vi "test2.vi"() -> ()   [LabVIEW 2009]
panel:
  out "time to read":dbl
  out "error out 2":errorcluster
  out "standard error 2":string
  out "standard output 2":string
  in  "command line 2":string
  out "time to create":dbl
  out "error out":errorcluster
  out "standard error":string
  out "standard output":string
  in  "command line":string
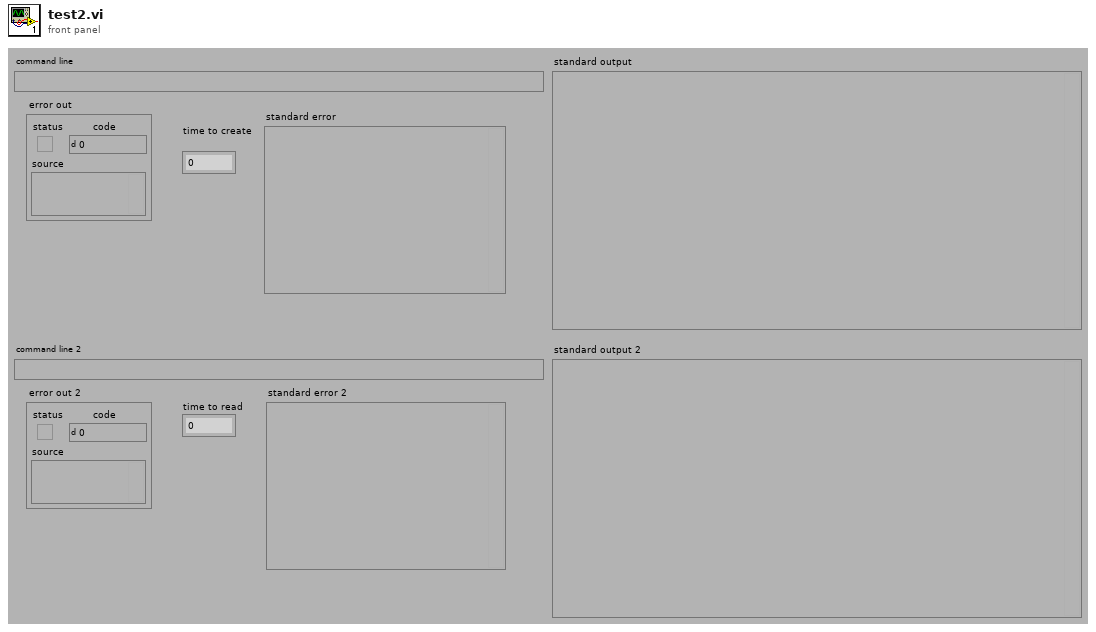
[diagram p1: front panel]
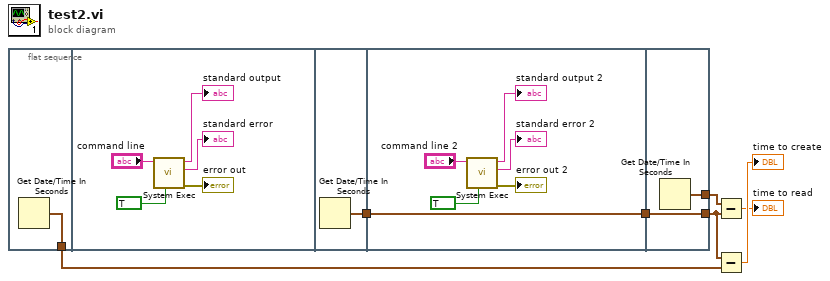
[diagram p0: block diagram]
diagram:
  n1 = flat-sequence {
    tunnel: [w8] -> w7
    tunnel: [w14] -> w5
    tunnel: w5 -> [w20]
    tunnel: [w20] -> w4
    tunnel: [w22] -> w2
    tunnel: w4 -> [w22]
    tunnel: [w21] -> w3
    frame #0 {
      n2 = Get Date/Time In Seconds() -> (seconds since 1Jan1904=w8:timestamp)
    }
    frame #1 {
      n3 = call <vilib>:"System Exec.vi"("run minimized? (F)"=TRUE, "command line"="command line") -> ("error out"=→"error out":errorcluster, "standard error"=→"standard error":string, "standard output"=→"standard output":string)  [unwired: 6 in, 1 out]
    }
    frame #2 {
      n4 = Get Date/Time In Seconds() -> (seconds since 1Jan1904=w14:timestamp)
    }
    frame #3 {
      n5 = call <vilib>:"System Exec.vi"("run minimized? (F)"=TRUE, "command line"="command line 2") -> ("error out"=→"error out 2":errorcluster, "standard error"=→"standard error 2":string, "standard output"=→"standard output 2":string)  [unwired: 6 in, 1 out]
    }
    frame #4 {
      n6 = Get Date/Time In Seconds() -> (seconds since 1Jan1904=w21:timestamp)
    }
  }
  n7 = Subtract(x=w3, y=w2) -> (x-y=→"time to read":dbl)
  n8 = Subtract(x=w2, y=w7) -> (x-y=→"time to create":dbl)
